vi "Rio_XY_Shutdown_(DONE).vi"(8 "error in (no error)":errorcluster) -> (0 "error out":errorcluster)   [LabVIEW 2017]
uses:
  motor_control_inputs.ctl
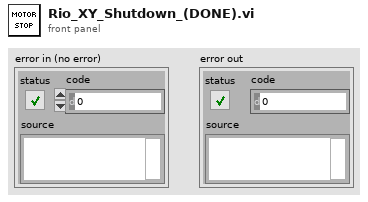
[diagram p1: front panel]
types:
  T1 = typedef "motor_control_inputs.ctl" = cluster{"X(t)/Y(f) Selection ":bool, "Duty Cycle (0-1) (X Control)":dbl, "Frequency [Hz] (Y Control)":dbl, "Direction (t:+, f:-)":bool}
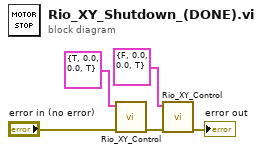
[diagram p0: block diagram]
diagram:
  n1 = call "Rio_XY_Control.vi"("Error In"="error in (no error)", "Input Cluster"=T1 {"X(t)/Y(f) Selection "=TRUE, "Duty Cycle (0-1) (X Control)"=0.0, "Frequency [Hz] (Y Control)"=0.0, "Direction (t:+, f:-)"=TRUE}) -> ("Error Out"=w3:errorcluster)  [unwired: 9 in]
  n2 = call "Rio_XY_Control.vi"("Error In"=w3, "Input Cluster"=T1 {"X(t)/Y(f) Selection "=FALSE, "Duty Cycle (0-1) (X Control)"=0.0, "Frequency [Hz] (Y Control)"=0.0, "Direction (t:+, f:-)"=TRUE}) -> ("Error Out"=→"error out":errorcluster)  [unwired: 9 in]
